vi "JSON CARGA.vi"(4 "time":u32, 5 "Potencia Fase 3":dbl, 6 "Corriente Fase 3":dbl, 7 "Corriente Fase 1":dbl, 8 "error in":errorcluster, 9 "Potencia Fase 2":dbl, 10 "Corriente Fase 2":dbl, 11 "Potencia Fase 1":dbl) -> (0 "error out":errorcluster, 3 "JSON Array out":refnum<class "JSON Array.lvclass">)   [LabVIEW 2015]
uses:
  <vilib>/addons/JSON API/JSON Array/Set JSON Array.vi
  <vilib>/addons/JSON API/JSON Array/JSON Array.lvclass
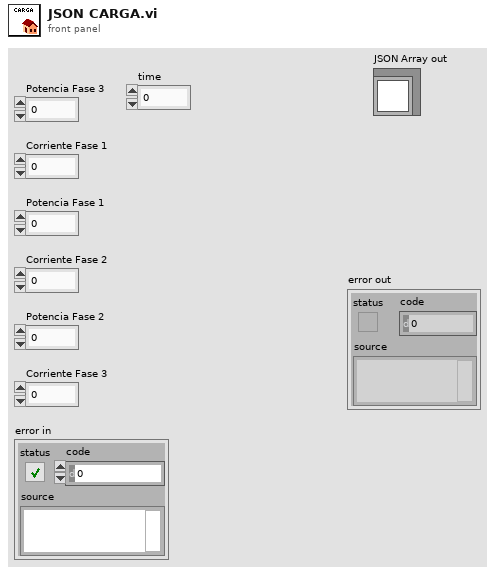
[diagram p1: front panel]
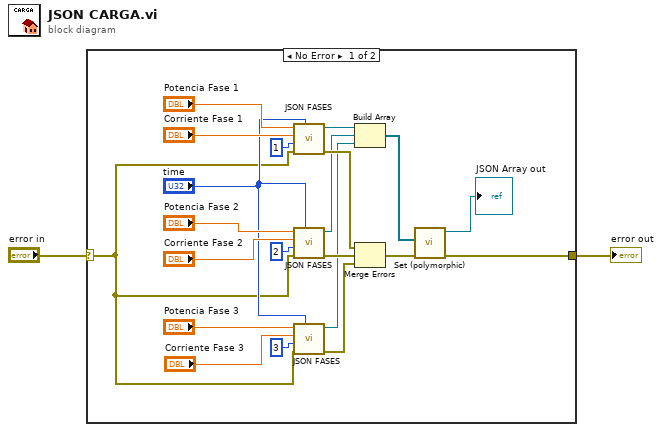
[diagram p0: block diagram]
diagram:
  n1 = case shown="No Error" "error in" {
    selector: "error in" -> [w3 w24]
    tunnel: [w4 w24] -> w1
    frame No Error {
      n2 = call "JSON FASES.vi"("time"="time", "error in"=w3, "Fase"=u32 1 ("Numeric"), "Corriente"="Corriente Fase 1", "Potencia"="Potencia Fase 1") -> ("error out"=w19:errorcluster, "JSON Object out"=w16:refnum<class "JSON Object.lvclass">)  [unwired: 5 in]
      n3 = call "JSON FASES.vi"("time"="time", "error in"=w3, "Fase"=u32 2, "Corriente"="Corriente Fase 2", "Potencia"="Potencia Fase 2") -> ("error out"=w20:errorcluster, "JSON Object out"=w18:refnum<class "JSON Object.lvclass">)  [unwired: 5 in]
      n4 = call "JSON FASES.vi"("time"="time", "error in"=w3, "Fase"=u32 3, "Corriente"="Corriente Fase 3", "Potencia"="Potencia Fase 3") -> ("error out"=w21:errorcluster, "JSON Object out"=w17:refnum<class "JSON Object.lvclass">)  [unwired: 5 in]
      n5 = Build Array(w16, w18, w17) -> (w23:refnum<class "JSON Object.lvclass">[])
      n6 = Merge Errors(w19, w20, w21) -> (w22:errorcluster)
      n7 = call-poly <vilib>:"Set (polymorphic).vi"("error in (no error)"=w22, "Array"=w23) -> ("error out"=w4:errorcluster, "JSON Array out"=→"JSON Array out":refnum<class "JSON Array.lvclass">)  [unwired: 8 in]
    }
    frame Error {
    }
  }
  "error out" <- w1
